vi "Measurement_Circle.vi"() -> ()   [LabVIEW 2016]
uses:
  Control/Coordinate.ctl
  <vilib>/Instr/_visa.llb/VISA Configure Serial Port (Instr).vi
  <vilib>/Instr/_visa.llb/VISA Flush IO Buffer Mask.ctl
panel:
  out "Lowest":string
  out "1 12":string
  out "1 11":string
  out "1 10":string
  out "1 9":string
  out "1 8":string
  out "1 7":string
  out "1 6":string
  out "1 5":string
  out "1 4":string
  out "1 3":string
  out "1 2":string
  out "1":string
  in  "File Name":string="tmp.txt"
  in  "Center":T1={"X"=968.59881, "Y"=892.69941, "Z"=0.0, "U"=0.0} {"U" format="%#.5g"; "X" format="%#.5g"; "Y" format="%#.5g"; "Z" format="%#.5g"}
  in  "VISA resource name":refnum<visa-resource-name>="COM4"
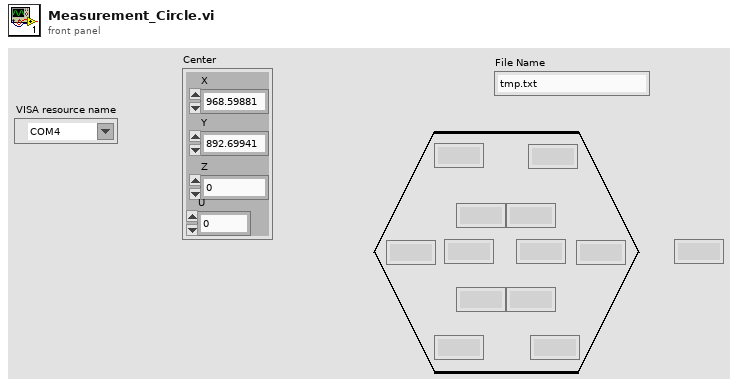
[diagram p1: front panel]
types:
  T1 = typedef "Coordinate.ctl" = cluster{"X":dbl, "Y":dbl, "Z":dbl, "U":dbl}
  T2 = typedef "VISA Flush IO Buffer Mask.ctl" = u16
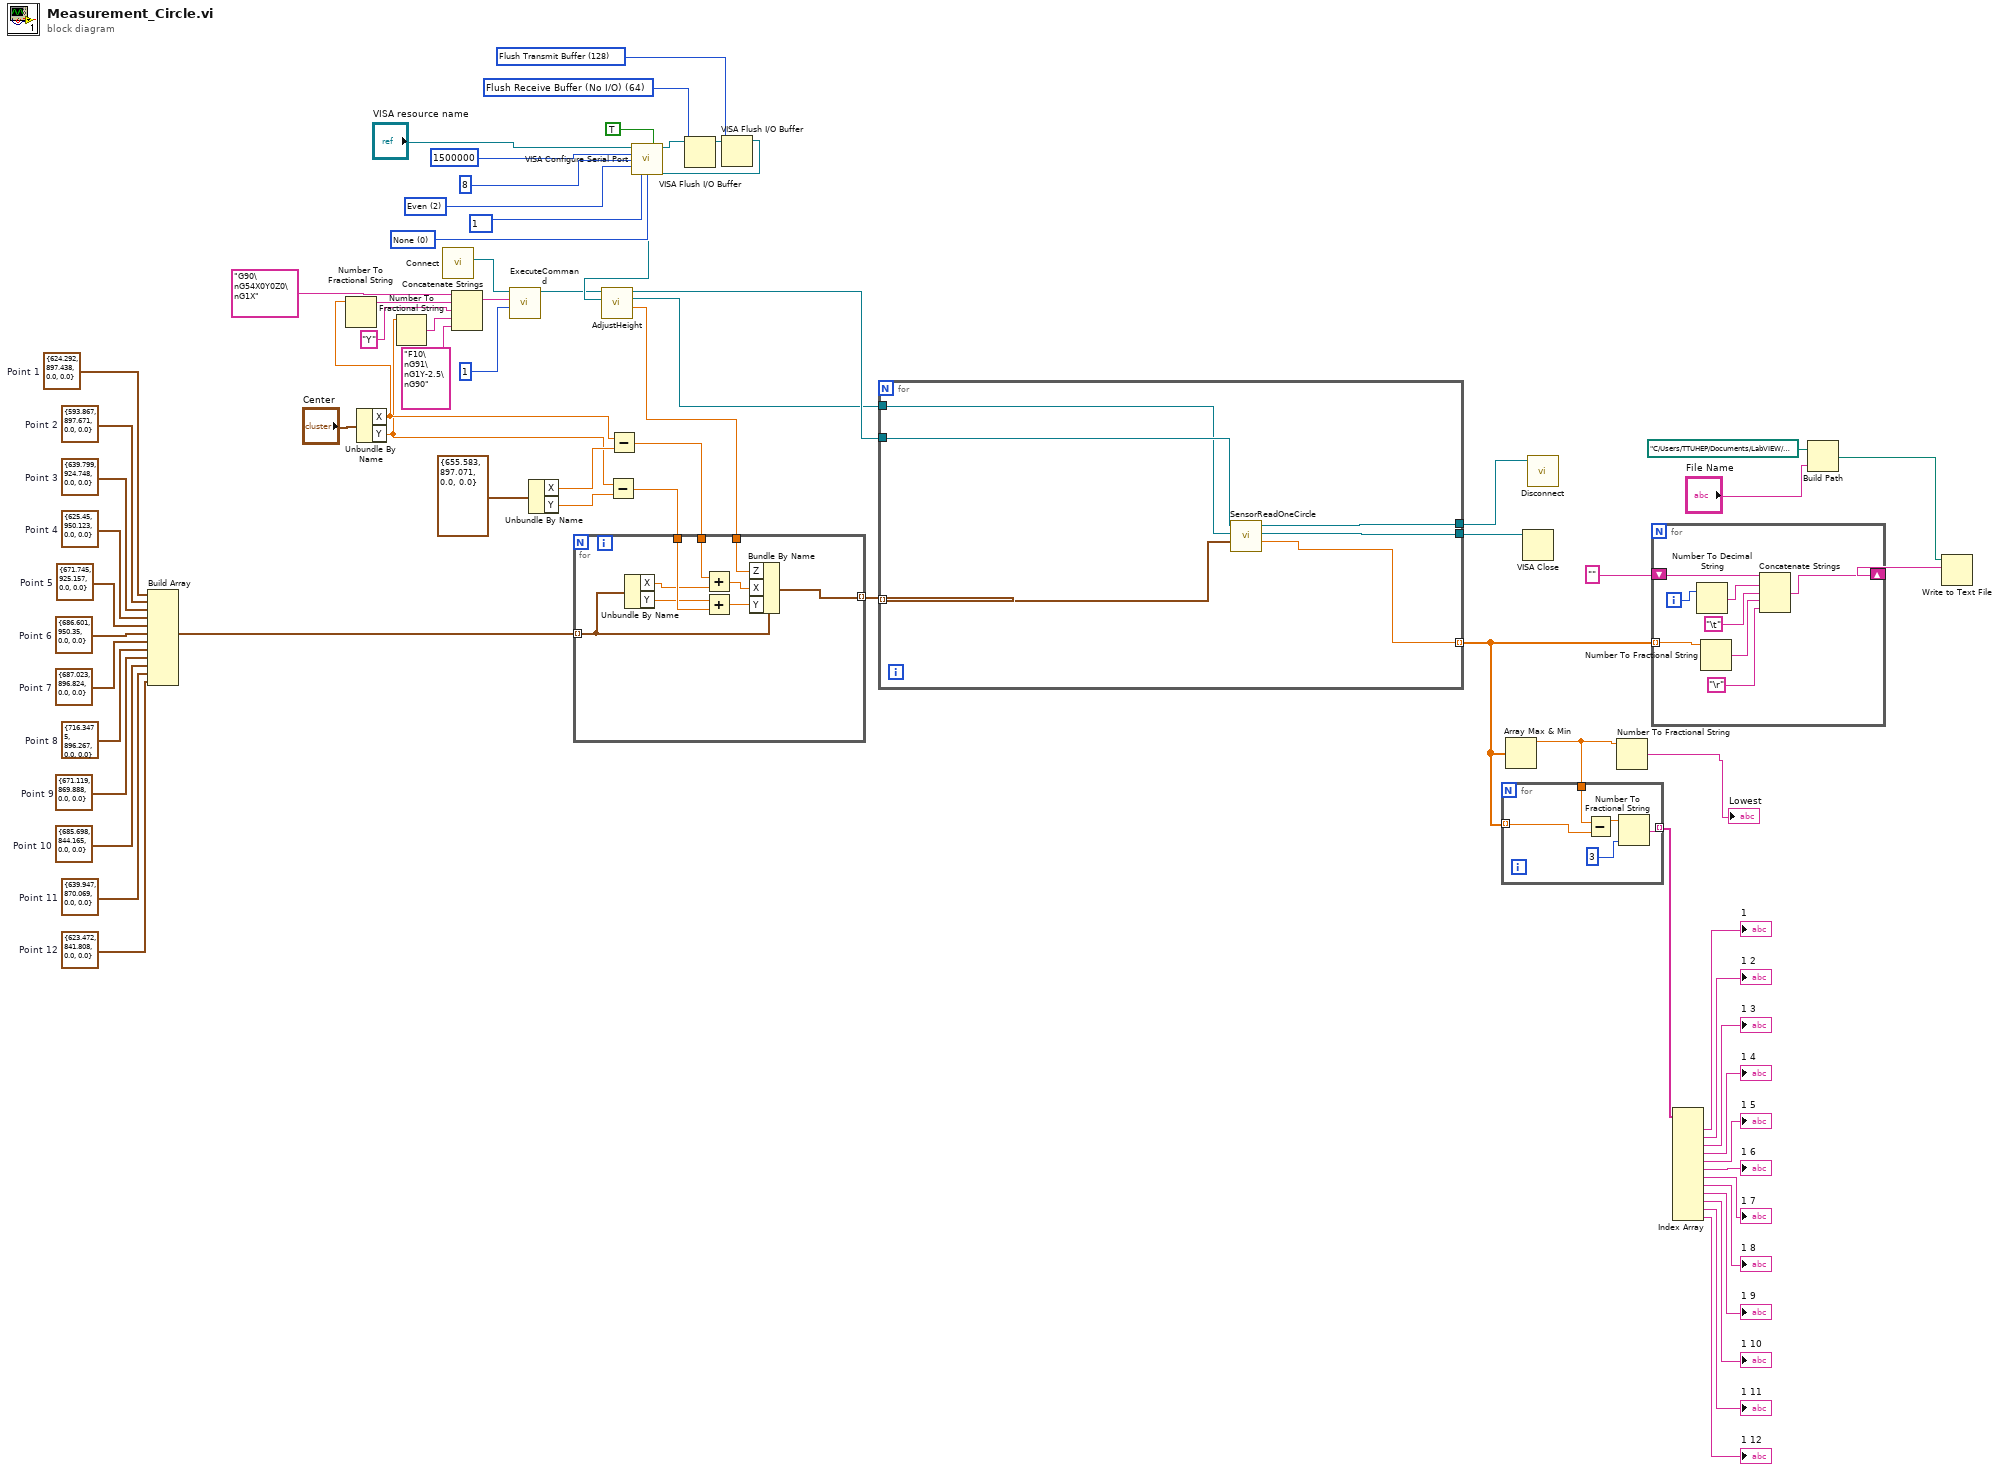
[diagram p0: block diagram]
diagram:
  w56 = u16 0 items=["None"=0, "XON/XOFF"=1, "RTS/CTS"=2, "DTR/DSR"=4] ("flow control")
  w55 = u16 10 items=["1"=10, "1.5"=15, "2.0"=20] ("stop bits")
  w54 = u16 2 items=["None", "Odd", "Even", "Mark", "Space"] ("parity")
  w38 = T2 128 items=["Flush Receive Buffer"=16, "Write Transmit Buffer to Device"=32, "Flush Receive Buffer (No I/O)"=64, "Flush Transmit Buffer"=128] ("Mask")
  w39 = T2 64 items=["Flush Receive Buffer"=16, "Write Transmit Buffer to Device"=32, "Flush Receive Buffer (No I/O)"=64, "Flush Transmit Buffer"=128] ("Mask")
  w62 = T1 {"X"=671.119, "Y"=869.888, "Z"=0.0, "U"=0.0}  # Point 9
  w66 = T1 {"X"=671.745, "Y"=925.157, "Z"=0.0, "U"=0.0}  # Point 5
  w59 = T1 {"X"=623.472, "Y"=841.808, "Z"=0.0, "U"=0.0}  # Point 12
  w63 = T1 {"X"=716.3475, "Y"=896.267, "Z"=0.0, "U"=0.0}  # Point 8
  w67 = T1 {"X"=625.45, "Y"=950.123, "Z"=0.0, "U"=0.0}  # Point 4
  w60 = T1 {"X"=639.947, "Y"=870.069, "Z"=0.0, "U"=0.0}  # Point 11
  w64 = T1 {"X"=687.023, "Y"=896.824, "Z"=0.0, "U"=0.0}  # Point 7
  w68 = T1 {"X"=639.799, "Y"=924.748, "Z"=0.0, "U"=0.0}  # Point 3
  w61 = T1 {"X"=685.698, "Y"=844.165, "Z"=0.0, "U"=0.0}  # Point 10
  w65 = T1 {"X"=686.601, "Y"=950.35, "Z"=0.0, "U"=0.0}  # Point 6
  w69 = T1 {"X"=593.867, "Y"=897.671, "Z"=0.0, "U"=0.0}  # Point 2
  w49 = T1 {"X"=624.292, "Y"=897.438, "Z"=0.0, "U"=0.0}  # Point 1
  n1 = Build Array(w49, w69, w68, w67, w66, w65, w64, w63, w62, w61, w60, w59) -> (w51:T1[])
  n2 = Unbundle By Name("Center") -> ("X"=w7:dbl, "Y"=w6:dbl)
  n3 = Number To Fractional String(number=w7) -> (F-format string=w8:string)  [unwired: 3 in]
  n4 = Number To Fractional String(number=w6) -> (F-format string=w4:string)  [unwired: 3 in]
  n5 = call "Connect.vi"() -> ("controller"=w34:refnum<k24>)  [unwired: 10 in, 1 out]
  n6 = Concatenate Strings("G90\nG54X0Y0Z0\nG1X", w8, "Y", w4, "F10\nG91\nG1Y-2.5\nG90") -> (w9:string)
  n7 = call "ExecuteCommand.vi"("taskId"=1, "Command Code"=w9, "controller in"=w34) -> ("controller out"=w12:refnum<k24>)  [unwired: 6 in, 2 out]
  n8 = Unbundle By Name(T1 {"X"=655.583, "Y"=897.071, "Z"=0.0, "U"=0.0} ("_Center")) -> ("X"=w48:dbl, "Y"=w47:dbl)
  n9 = Subtract(x=w6, y=w47) -> (x-y=w45:dbl)
  n10 = Subtract(x=w7, y=w48) -> (x-y=w46:dbl)
  n11 = call-poly "VISA Configure Serial Port"("VISA resource name"="VISA resource name", "Enable Termination\nChar (T)"=TRUE, "baud rate (9600)"=u32 1500000 ("baud rate"), "data bits (8)"=u16 8 ("data bits"), "parity (0:none)"=w54, "stop bits (10: 1 bit)"=w55, "flow control (0:none)"=w56) -> ("VISA resource name out"=w41:refnum<visa-resource-name>)  [unwired: 7 in, 1 out]
  n12 = VISA Flush I/O Buffer(VISA resource name=w41, mask (16)=w39) -> (VISA resource name out=w40:refnum<visa-resource-name>)  [unwired: 1 in, 1 out]
  n13 = VISA Flush I/O Buffer(VISA resource name=w40, mask (16)=w38) -> (VISA resource name out=w14:refnum<visa-resource-name>)  [unwired: 1 in, 1 out]
  n14 = call "AdjustHeight.vi"("VISA resource name"=w14, 11:w12) -> ("Z Position"=w11:dbl, "VISA resource name out"=w13:refnum<visa-resource-name>, "controller out"=w15:refnum<k24>)  [unwired: 6 in, 1 out]
  n15 = for {
    tunnel: w51 -> [w78] mode=indexing
    tunnel: w46 -> [w75]
    tunnel: w45 -> [w74]
    tunnel: [w71] -> w44 mode=indexing
    tunnel: w11 -> [w70]
    n16 = Unbundle By Name(w78) -> ("X"=w72:dbl, "Y"=w73:dbl)
    n17 = Add(x=w75, y=w72) -> (x+y=w76:dbl)
    n18 = Add(x=w73, y=w74) -> (x+y=w77:dbl)
    n19 = Bundle By Name(cluster=w78, "Z"=w70, "X"=w76, "Y"=w77) -> (w71:T1)
  }
  n20 = for {
    tunnel: w44 -> [w84] mode=indexing
    tunnel: w15 -> [w83]
    tunnel: w13 -> [w82]
    tunnel: [w81] -> w29 mode=indexing
    tunnel: [w80] -> w32
    tunnel: [w79] -> w31
    n21 = call "SensorReadOneCircle.vi"("controller"=w83, "VISA resource name"=w82, "StartPoint"=w84) -> ("controller out"=w80:refnum<k24>, "VISA resource name out"=w79:refnum<visa-resource-name>, "AverageReading"=w81:dbl)  [unwired: 4 in, 1 out]
  }
  n22 = Array Max & Min(array=w29) -> (max value=w2:dbl)  [unwired: 3 out]
  n23 = for {
    tunnel: w29 -> [w89] mode=indexing
    tunnel: w2 -> [w88]
    tunnel: [w87] -> w28 mode=indexing
    n24 = Subtract(x=w88, y=w89) -> (x-y=w86:dbl)
    n25 = Number To Fractional String(number=w86, precision (6)=3) -> (F-format string=w87:string)  [unwired: 2 in]
  }
  n26 = VISA Close(VISA resource name=w31) -> ()  [unwired: 1 in, 1 out]
  n27 = call "Disconnect.vi"("controller"=w32) -> ()  [unwired: 10 in, 1 out]
  n28 = Number To Fractional String(number=w2) -> (F-format string=→"Lowest":string)  [unwired: 3 in]
  n29 = for {
    tunnel: w29 -> [w97] mode=indexing
    shift-right: [w95] -> w42
    shift-left: "" -> [w96]
    i -> [w94]
    n30 = Number To Decimal String(number=w94) -> (decimal integer string=w93:string)  [unwired: 1 in]
    n31 = Number To Fractional String(number=w97) -> (F-format string=w91:string)  [unwired: 3 in]
    n32 = Concatenate Strings(w96, w93, "\t", w91, "\r") -> (w95:string)
  }
  n33 = Index Array(array=w28) -> (element #1=→"1":string, element #2=→"1 2":string, element #3=→"1 3":string, element #4=→"1 4":string, element #5=→"1 5":string, element #6=→"1 6":string, element #7=→"1 7":string, element #8=→"1 8":string, element #9=→"1 9":string, element #10=→"1 10":string, element #11=→"1 11":string, element #12=→"1 12":string)  [unwired: 12 in]
  n34 = Build Path(base path=path "C:/Users/TTUHEP/Documents/LabVIEW/Data/Center", name or relative path="File Name") -> (appended path=w35:path)
  n35 = Write to Text File(file (use dialog)=w35, text=w42) -> ()  [unwired: 2 in, 3 out]
